vi "drive train control.vi"(5 "Max":dbl, 6 "take motor input":bool, 7 "Square Inputs":bool, 9 "input 1":dbl, 10 "input 2":dbl) -> ()   [LabVIEW 2018]
panel:
  out "?":dbl
  out "?":dbl
  out "?":dbl
  out "?":dbl
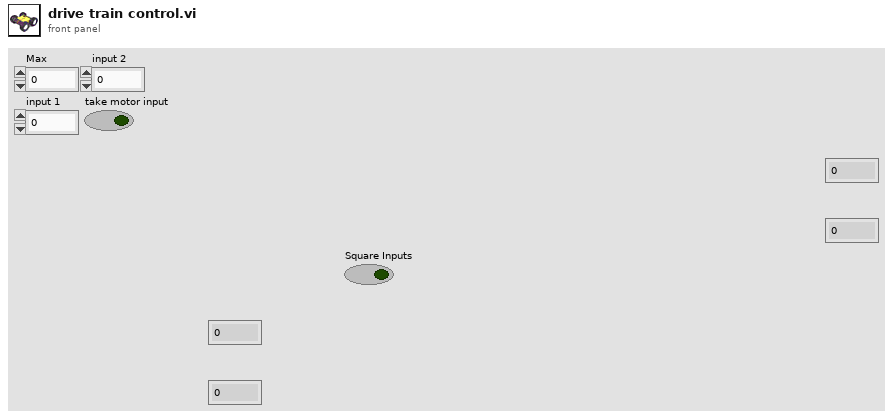
[diagram p1: front panel]
types:
  T1 = typedef "WPI_MotorControlDeviceRef.ctl" = cluster{"DeviceStatus":errorcluster, "Type":T2, "PWM":cluster{"PWM Channel":T3, "DeadBand":T4}, "CAN":cluster{"Device Number":u8, "SetOutput VI Ref":variant, "GetOutput VI Ref":variant, "Enable VI Ref":variant, "Disable VI Ref":variant, "Data":variant}, "Invert":bool, "DIO PWM":cluster{"PWM \"Enable\" Channel":T3, "DIOChannel":T5, "PWM Rate":dbl}}
  T2 = typedef "WPI_MotorControlType.ctl" = enum16{"PWM", "CAN", "DIO PWM"}
  T3 = typedef "FPGA_DIOPWMChannel.ctl" = enum8{"PWM 0", "PWM 1", "PWM 2", "PWM 3", "PWM 4", "PWM 5", "PWM 6", "PWM 7", "PWM 8", "PWM 9", "PWM MXP 0", "PWM MXP 1", "PWM MXP 2", "PWM MXP 3", "PWM MXP 4", "PWM MXP 5", "PWM MXP 6", "PWM MXP 7", "PWM MXP 8", "PWM MXP 9", "Invalid"}
  T4 = typedef "WPI_PWMDeadband.ctl" = cluster{"Name":string, "maxPositivePwm":i32, "minPositivePwm":i32, "centerPwm":i32, "maxNegativePwm":i32, "minNegativePwm":i32, "angularRange":u16}
  T5 = typedef "FPGA_DIOChannel.ctl" = enum8{"DIO 0", "DIO 1", "DIO 2", "DIO 3", "DIO 4", "DIO 5", "DIO 6", "DIO 7", "DIO 8", "DIO 9", "DIO MXP 0", "DIO MXP 1", "DIO MXP 2", "DIO MXP 3", "DIO MXP 4", "DIO MXP 5", "DIO MXP 6", "DIO MXP 7", "DIO MXP 8", "DIO MXP 9", "DIO MXP 10", "DIO MXP 11", "DIO MXP 12", "DIO MXP 13", "DIO MXP 14", "DIO MXP 15", "SPI Port CS1", "SPI Port CS2", "SPI Port CS3", "SPI Port MISO", "SPI Port MOSI", "Invalid"}
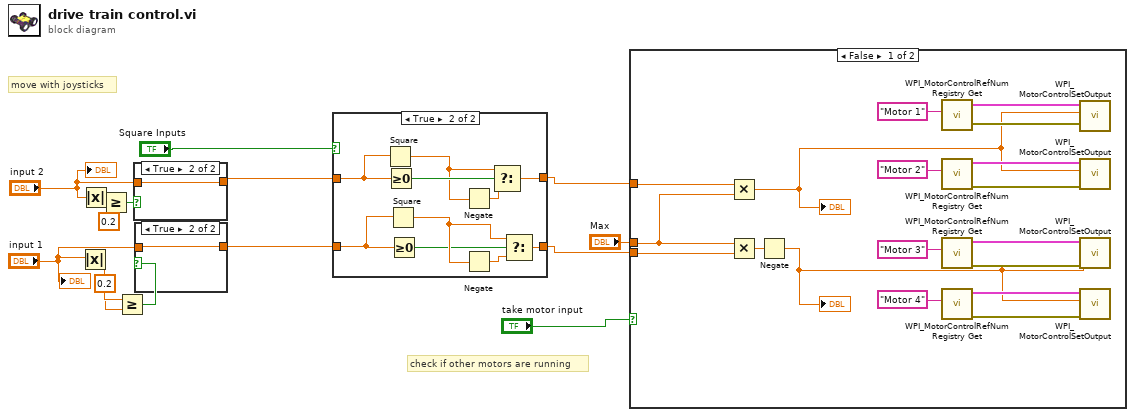
[diagram p0: block diagram]
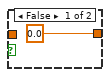
[diagram p3: hidden frame]
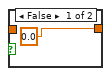
[diagram p4: hidden frame]
diagram:
  # "check if other motors are running"
  # "move with joysticks"
  n1 = Absolute Value(x="input 1") -> (abs(x)=w11:dbl)
  n2 = Absolute Value(x="input 2") -> (abs(x)=w12:dbl)
  n3 = Greater Or Equal?(x=w12, y=0.2) -> (x >= y?=w13:bool)
  n4 = Greater Or Equal?(x=w11, y=0.2) -> (x >= y?=w10:bool)
  n5 = case shown="True" w13 {
    tunnel: [0.0 ("upper limit") w17] -> w8
    tunnel: "input 2" -> [_ w17]
    frame False {
    }
    frame True {
    }
  }
  n6 = case shown="True" w10 {
    tunnel: [0.0 ("upper limit") w19] -> w7
    tunnel: "input 1" -> [_ w19]
    frame False {
    }
    frame True {
    }
  }
  n7 = case shown="True" "Square Inputs" {
    tunnel: w8 -> [w21 w31]
    tunnel: [w21 w27] -> w5
    tunnel: w7 -> [w20 w26]
    tunnel: [w20 w25] -> w6
    frame False {
    }
    frame True {
      n8 = Square(x=w31) -> (x^2=w29:dbl)
      n9 = Greater Or Equal To 0?(x=w31) -> (x >= 0?=w30:bool)
      n10 = Square(x=w26) -> (x^2=w24:dbl)
      n11 = Greater Or Equal To 0?(x=w26) -> (x >= 0?=w22:bool)
      n12 = Negate(x=w29) -> (-x=w28:dbl)
      n13 = Negate(x=w24) -> (-x=w23:dbl)
      n14 = Select(t=w29, s=w30, f=w28) -> (s? t:f=w27:dbl)
      n15 = Select(t=w24, s=w22, f=w23) -> (s? t:f=w25:dbl)
    }
  }
  n16 = case shown="False" "take motor input" {
    tunnel: "Max" -> [w34 _]
    tunnel: w5 -> [w32 _]
    tunnel: w6 -> [w33 _]
    frame False {
      n17 = Multiply(x=w32, y=w34) -> (x*y=w35:dbl)
      "?" <- w35
      n18 = Multiply(x=w34, y=w33) -> (x*y=w38:dbl)
      n19 = Negate(x=w38) -> (-x=w36:dbl)
      "?" <- w36
      n20 = call <vilib>:"WPI_MotorControlRefNum Registry Get.vi"("refnum name"="Motor 1") -> ("error out"=w49:errorcluster, "MotorControlDevRef"=w48:T1)  [unwired: 9 in]
      n21 = call <vilib>:"WPI_MotorControlRefNum Registry Get.vi"("refnum name"="Motor 2") -> ("error out"=w46:errorcluster, "MotorControlDevRef"=w47:T1)  [unwired: 9 in]
      n22 = call <vilib>:"WPI_MotorControlRefNum Registry Get.vi"("refnum name"="Motor 3") -> ("error out"=w43:errorcluster, "MotorControlDevRef"=w42:T1)  [unwired: 9 in]
      n23 = call <vilib>:"WPI_MotorControlRefNum Registry Get.vi"("refnum name"="Motor 4") -> ("error out"=w40:errorcluster, "MotorControlDevRef"=w41:T1)  [unwired: 9 in]
      n24 = call <vilib>:"WPI_MotorControlSetOutput.vi"("error in (no error)"=w49, "Output"=w35, "MotorControlDevRef"=w48) -> ()  [unwired: 6 in, 3 out]
      n25 = call <vilib>:"WPI_MotorControlSetOutput.vi"("error in (no error)"=w46, "Output"=w35, "MotorControlDevRef"=w47) -> ()  [unwired: 6 in, 3 out]
      n26 = call <vilib>:"WPI_MotorControlSetOutput.vi"("error in (no error)"=w43, "Output"=w36, "MotorControlDevRef"=w42) -> ()  [unwired: 6 in, 3 out]
      n27 = call <vilib>:"WPI_MotorControlSetOutput.vi"("error in (no error)"=w40, "Output"=w36, "MotorControlDevRef"=w41) -> ()  [unwired: 6 in, 3 out]
    }
    frame True {
    }
  }
  "?" <- "input 1"
  "?" <- "input 2"
